vi "HEWH Find Qr Indexes.vi"(0 "Watt Hours (String)":string[](array[string]), 5 "UE":i32[](array[numeric]), 7 "LE":i32[](array[numeric]), 9 "Comp":i32[](array[numeric]), 11 "Error In":errorcluster) -> (4 "Qr (BTU)":dbl, 6 "First Recovery End":i32, 10 "First Recovery Start":i32, 15 "Error Out":errorcluster)   [LabVIEW 2016]
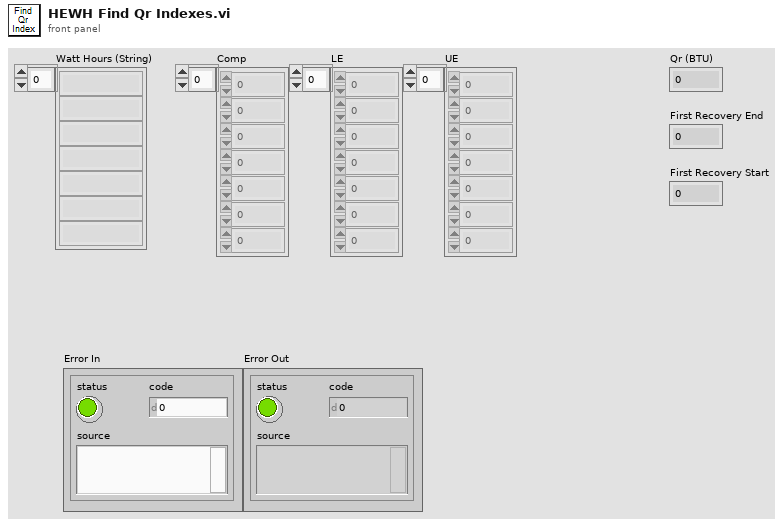
[diagram p1: front panel]
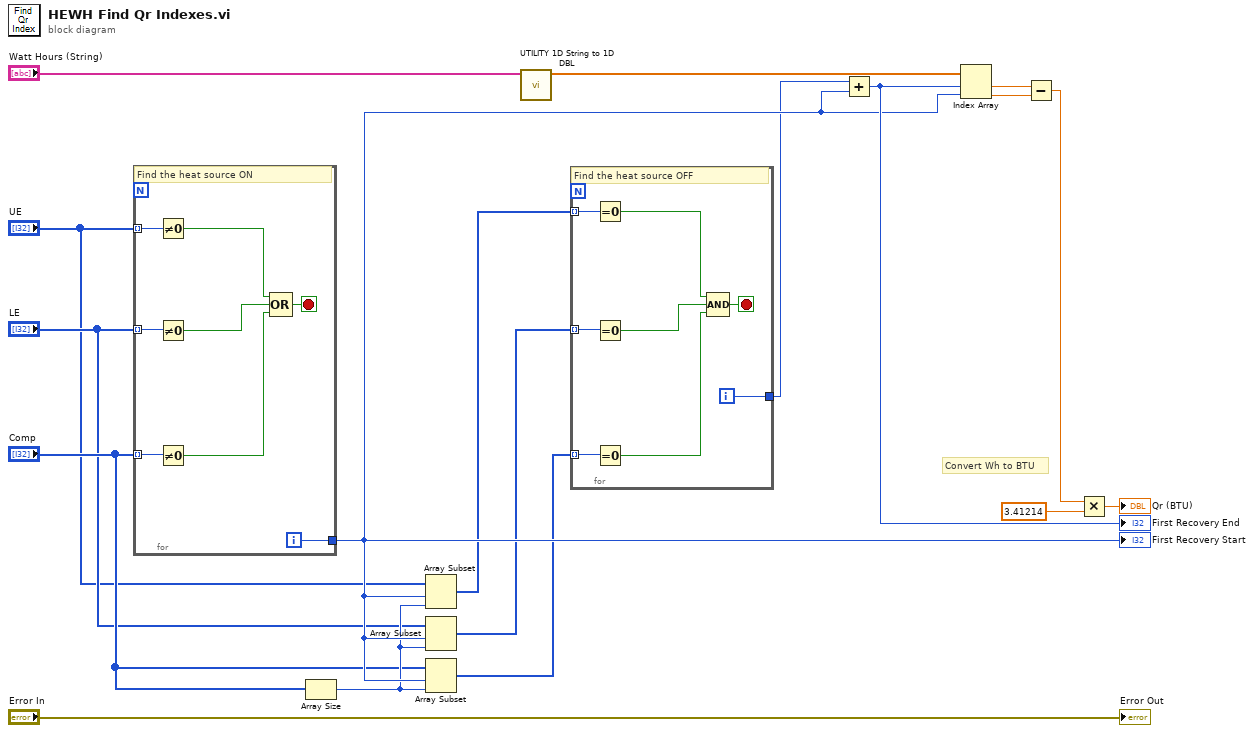
[diagram p0: block diagram]
diagram:
  # "Convert Wh to BTU"
  n1 = for {
    tunnel: "UE" -> [w26] mode=indexing
    tunnel: "LE" -> [w24] mode=indexing
    tunnel: "Comp" -> [w25] mode=indexing
    tunnel: [w19] -> w12
    i -> [w19]
    stop <- w20 stop-if-true
    # "Find the heat source ON"
    n2 = Not Equal To 0?(x=w26) -> (x != 0?=w23:bool)
    n3 = Not Equal To 0?(x=w24) -> (x != 0?=w22:bool)
    n4 = Not Equal To 0?(x=w25) -> (x != 0?=w21:bool)
    n5 = Compound Arithmetic op=OR(w23, w22, w21) -> (w20:bool)
  }
  "First Recovery Start" <- w12
  n6 = Array Size(array="Comp") -> (size(s)=w5:i32)
  n7 = Array Subset(array="UE", index=w12, length=w5) -> (w6:i32[])
  n8 = Array Subset(array="LE", index=w12, length=w5) -> (w7:i32[])
  n9 = Array Subset(array="Comp", index=w12, length=w5) -> (w8:i32[])
  n10 = call "UTILITY 1D String to 1D DBL.vi"("Save Data"="Watt Hours (String)") -> ("DBL"=w10:dbl[])  [unwired: 10 in]
  n11 = for {
    tunnel: w6 -> [w34] mode=indexing
    tunnel: w7 -> [w32] mode=indexing
    tunnel: w8 -> [w33] mode=indexing
    tunnel: [w27] -> w11
    i -> [w27]
    stop <- w28 stop-if-true
    # "Find the heat source OFF"
    n12 = Equal To 0?(x=w34) -> (x = 0?=w31:bool)
    n13 = Equal To 0?(x=w32) -> (x = 0?=w30:bool)
    n14 = Equal To 0?(x=w33) -> (x = 0?=w29:bool)
    n15 = Compound Arithmetic op=AND(w31, w30, w29) -> (w28:bool)
  }
  n16 = Add(x=w11, y=w12) -> (x+y=w13:i32)
  "First Recovery End" <- w13
  n17 = Index Array(array=w10, index #1=w13, index #2=w12) -> (element #1=w14:dbl, element #2=w15:dbl)
  n18 = Subtract(x=w14, y=w15) -> (x-y=w16:dbl)
  n19 = Multiply(x=w16, y=3.41214) -> (x*y=→"Qr (BTU)":dbl)
  "Error Out" <- "Error In"
